vi "UpdatePosition.vi"(0 "MissionTime":dbl, 5 "possible location":T1, 7 "old location":cluster{dbl, i32, i32, i32}, 9 "current radius^2":dbl, 11 "starting radius^2":dbl) -> (8 "new location":cluster{"MissionTime":dbl, i32, i32, i32}, 10 "new radius^2":dbl, 15 "updated pos?":bool)   [LabVIEW 2012]
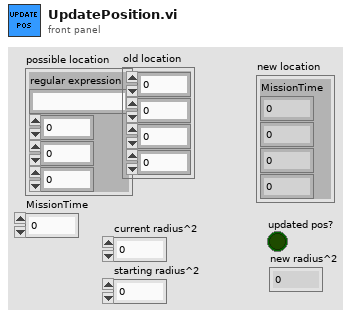
[diagram p1: front panel]
types:
  T1 = cluster{"regular expression":string, i32, i32, i32}
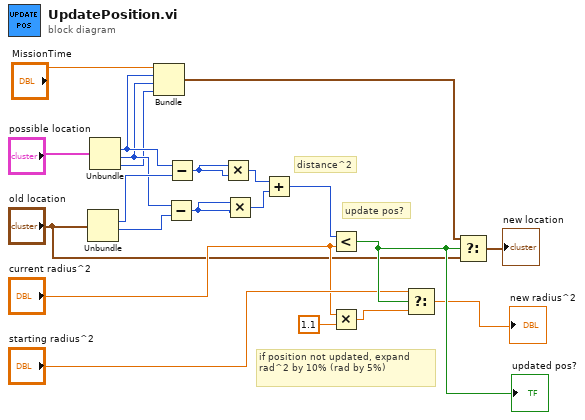
[diagram p0: block diagram]
diagram:
  # "if position not updated, expand rad^2 by 10% (rad by 5%)"
  # "update pos?"
  # "distance^2"
  n1 = Unbundle("old location") -> (w20:i32, w19:i32)  [unwired: 2 out]
  n2 = Unbundle("possible location") -> (w6:i32, w5:i32, w4:i32)  [unwired: 1 out]
  n3 = Bundle("MissionTime"="MissionTime", w6, w5, w4) -> (w3:cluster{"MissionTime":dbl, i32, i32, i32})  [unwired: 1 in]
  n4 = Subtract(x=w5, y=w19) -> (x-y=w17:i32)
  n5 = Subtract(x=w6, y=w20) -> (x-y=w18:i32)
  n6 = Multiply(x=w18, y=w18) -> (x*y=w16:i32)
  n7 = Multiply(x=w17, y=w17) -> (x*y=w15:i32)
  n8 = Add(x=w16, y=w15) -> (x+y=w14:i32)
  n9 = Less?(x=w14, y="current radius^2") -> (x < y?=w13:bool)
  "updated pos?" <- w13
  n10 = Multiply(x="current radius^2", y=1.1) -> (x*y=w9:dbl)
  n11 = Select(t="starting radius^2", s=w13, f=w9) -> (s? t:f=→"new radius^2":dbl)
  n12 = Select(t=w3, s=w13, f="old location") -> (s? t:f=→"new location":cluster{"MissionTime":dbl, i32, i32, i32})
